vi "Time.vi"(8 "error in (no error)":errorcluster, 10 "Control In":T1, 11 "CAD Dispense in":refnum<class "CAD Dispense.lvclass">) -> (0 "error out":errorcluster, 1 "Timing Data":i32[](array[numeric]), 2 "Control Out":T1, 3 "CAD Dispense out":refnum<class "CAD Dispense.lvclass">)   [LabVIEW 2020, in "CAD Dispense.lvclass"]
uses:
  CAD Dispense.lvclass
  Controller/Controllers.ctl
  Controller/I-O/I-O.lvclass
  Controller/Dispenser/Dispenser.lvclass
  C:/Program Files (x86)/Aerotech/A3200/LabVIEW/2010/Bin/Aerotech.A3200.dll
  Program Files (x86)/Aerotech/A3200/LabVIEW/2010/Bin/Aerotech.A3200.dll
  CAD Dispense.lvclass/CAD Dispense.ctl
  Controller/Motion/Motion.lvclass
  Controller/Motion/A3200/A3200.lvclass
  Controller/Controller.lvclass
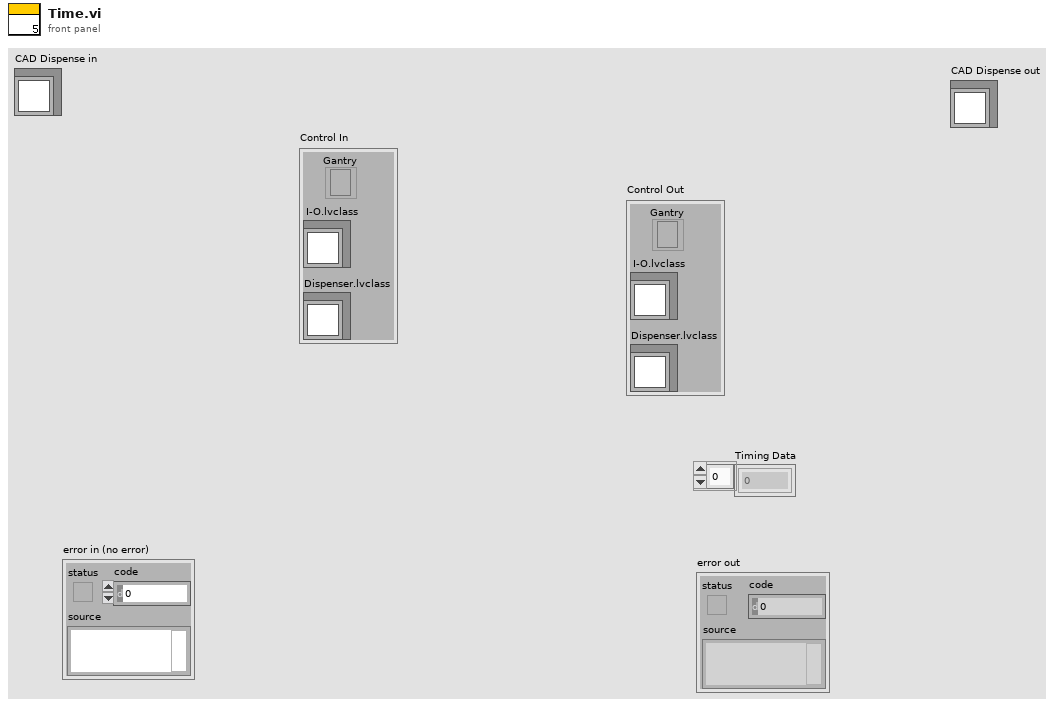
[diagram p1: front panel]
types:
  T1 = typedef "Controller.lvclass/Controllers.ctl" = cluster{"I-O.lvclass":refnum<class "I-O.lvclass">, "Dispenser.lvclass":refnum<class "Dispenser.lvclass">, "Gantry":refnum<k24>}
  T2 = cluster{"Motion":dbl[][], "Center":dbl[], "Circle?":bool, "CW/CCW":dbl}[]
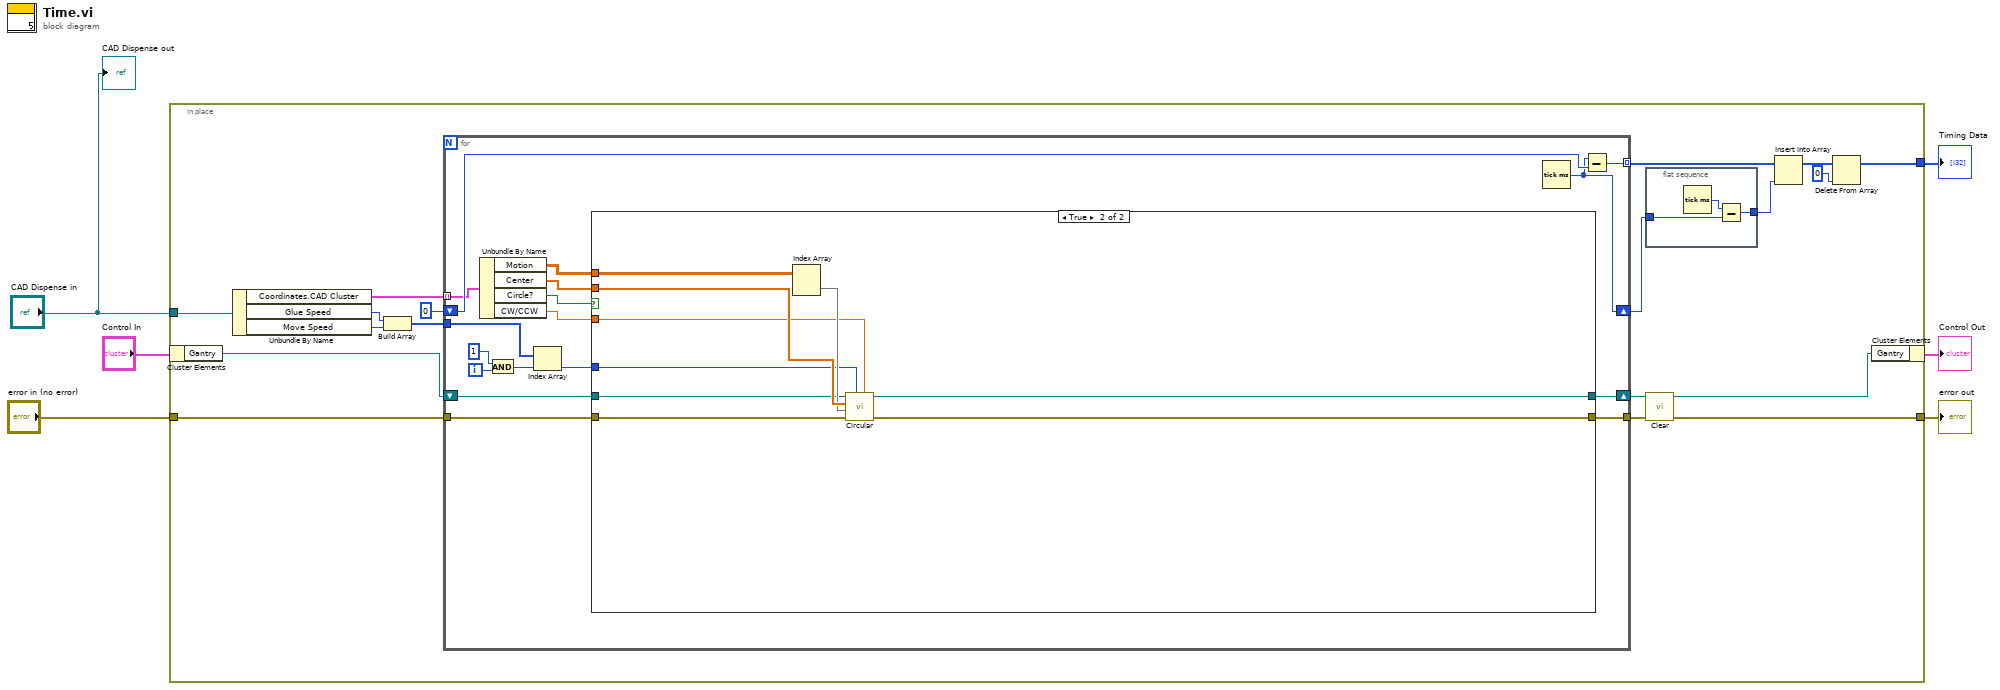
[diagram p0: block diagram]
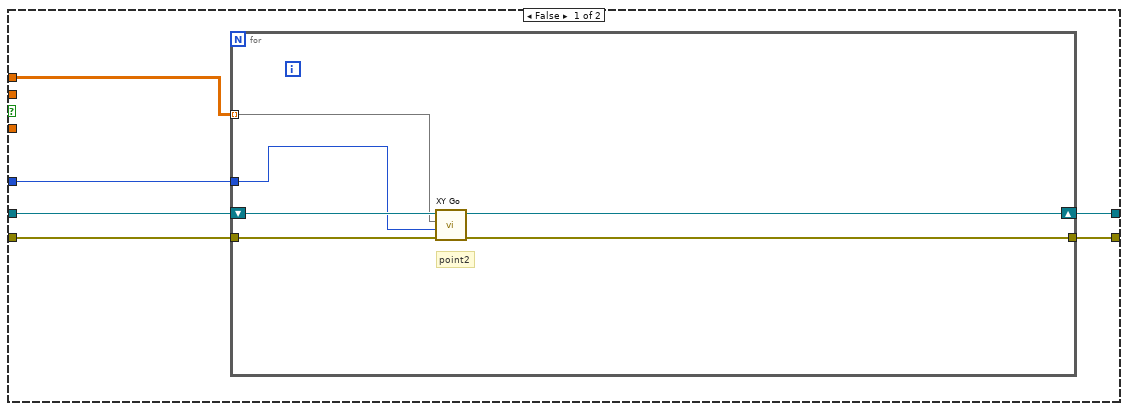
[diagram p2: hidden frame]
diagram:
  n1 = in-place {
    in-place-border: "CAD Dispense in" -> [w24]
    in-place-border: [w13] -> w5
    in-place-border: "error in (no error)" -> [w9]
    in-place-border: [w8] -> w1
    n2 = in-place-cluster #1("Control In") -> ("Gantry"=w11:refnum<k24>)
    n3 = Unbundle By Name(w24) -> ("Coordinates.CAD Cluster"=w14:T2, "Glue Speed"=w16:i32, "Move Speed"=w15:i32)
    n4 = Build Array(w16, w15) -> (w17:i32[])
    n5 = for {
      shift-right: [w39] -> w18
      shift-left: u32 0 ("millisecond timer value") -> [w42]
      tunnel: [w41] -> w20 mode=indexing
      tunnel: w14 -> [w37] mode=indexing
      tunnel: w17 -> [w33]
      shift-right: [w31] -> w12
      shift-left: w11 -> [w30]
      tunnel: w9 -> [w29]
      tunnel: [w28] -> w7
      i -> [w43]
      n6 = Unbundle By Name(w37) -> ("Motion"=w36:dbl[][], "Center"=w35:dbl[], "Circle?"=w34:bool, "CW/CCW"=w32:dbl)
      n7 = And(x=1, y=w43) -> (x .and. y?=w40:i32)
      n8 = Index Array(array=w33, index=w40) -> (element=w38:i32)
      n9 = case shown="True" w34 {
        tunnel: w38 -> [w50 w57]
        tunnel: w36 -> [w47 w65]
        tunnel: w35 -> [_ w64]
        tunnel: w32 -> [_ w58]
        tunnel: [w49 w62] -> w31
        tunnel: w30 -> [w46 w61]
        tunnel: w29 -> [w48 w60]
        tunnel: [w45 w59] -> w28
        frame False {
          n10 = for {
            tunnel: w50 -> [w54]
            shift-right: [w52] -> w49
            shift-left: w46 -> [w55]
            tunnel: w48 -> [w56]
            tunnel: w47 -> [w53] mode=indexing
            tunnel: [w51] -> w45
            # "point2"
            n11 = call "XY Go.vi"("error in (no error)"=w56, "Speed"=w54, "XY"=w53, "Gantry 2"=w55) -> ("error out"=w51:errorcluster, "Gantry 3"=w52:refnum<k24>)  [unwired: 6 in]
          }
        }
        frame True {
          n12 = Index Array(array=w65) -> (element=w63:dbl[])  [unwired: 2 in]
          n13 = call "Circular.vi"("Direction"=w58, "Speed"=w57, "error in (no error)"=w60, "XY End"=w63, "XY Center"=w64, "Gantry 2"=w61) -> ("error out"=w59:errorcluster, "Gantry 3"=w62:refnum<k24>)  [unwired: 4 in]
        }
      }
      n14 = Tick Count (ms)() -> (millisecond timer value=w39:u32)
      n15 = Subtract(x=w39, y=w42) -> (x-y=w41:u32)
    }
    n16 = flat-sequence {
      tunnel: [w26] -> w21
      tunnel: w18 -> [w25]
      frame #0 {
        n17 = Tick Count (ms)() -> (millisecond timer value=w27:u32)
        n18 = Subtract(x=w27, y=w25) -> (x-y=w26:u32)
      }
    }
    n19 = call "Clear.vi"("error in (no error)"=w7, "Gantry 2"=w12) -> ("error out"=w8:errorcluster, "Gantry 3"=w10:refnum<k24>)  [unwired: 8 in]
    n20 = Insert Into Array(array=w20, new element=w21) -> (w19:u32[])  [unwired: 1 in]
    n21 = Delete From Array(array=w19, index=0) -> (array with subset deleted=w13:u32[])  [unwired: 1 in, 1 out]
    n22 = in-place-cluster #1("Gantry"=w10) -> (→"Control Out":T1)
  }
  "error out" <- w1
  "Timing Data" <- w5
  "CAD Dispense out" <- "CAD Dispense in"
